vi "Keithley 6514 Read Math Result.vi"(0 "Resource In":refnum<visa-resource-name>, 1 "Check For SCPI Errors? (T)":bool=TRUE, 7 "read source (Math Result:0)":u16(ring) items=["Math Result", "Buffer Statistic"], 11 "error in (no error)":T1) -> (4 "Resource Out (dupl)":refnum<visa-resource-name>, 8 "result":dbl format="%.6e", 15 "error out":T1)   [LabVIEW 2014, in "KE6514Driver.lvlib"]
doc: "This VI is used to read the results of the selected calculation. The calculations are configured using the Math, or Buffer Math VI's. \n\nThese calculations do not show up in the other read VI's.\n\nRead Source:\n0 = Math\n1 = Buffer Math"
uses:
  KE6514Driver.lvlib
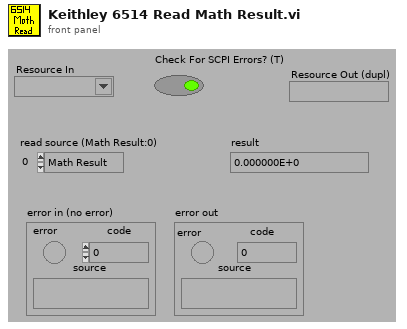
[diagram p1: front panel]
types:
  T1 = cluster{"error":bool, "code":i32, "source":string}
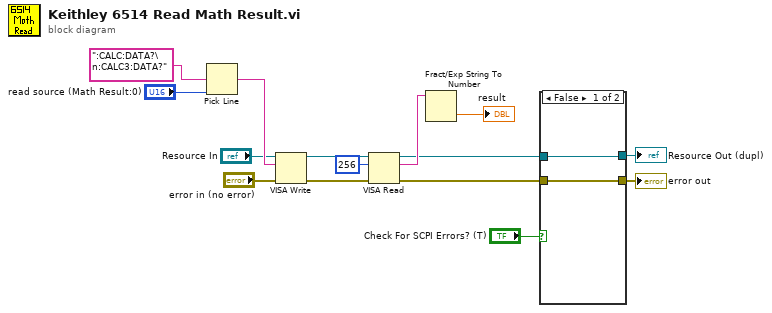
[diagram p0: block diagram]
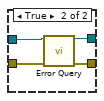
[diagram p2: hidden frame]
diagram:
  n1 = Pick Line(multi-line string=":CALC:DATA?\n:CALC3:DATA?", line index="read source (Math Result:0)") -> (output string=w8:string)  [unwired: 1 in]
  n2 = VISA Write(VISA resource name="Resource In", write buffer=w8, error in (no error)="error in (no error)") -> (VISA resource name out=w10:refnum<visa-resource-name>, error out=w11:errorcluster)  [unwired: 1 out]
  n3 = VISA Read(VISA resource name=w10, byte count=u32 256, error in (no error)=w11) -> (VISA resource name out=w4:refnum<visa-resource-name>, read buffer=w6:string, error out=w3:errorcluster)  [unwired: 1 out]
  n4 = Fract/Exp String To Number(string=w6) -> (number=→"result":dbl)  [unwired: 3 in, 1 out]
  n5 = case shown="False" "Check For SCPI Errors? (T)" {
    tunnel: w4 -> [w17 w20]
    tunnel: w3 -> [w16 w21]
    tunnel: [w16 w19] -> w1
    tunnel: [w17 w18] -> w2
    frame False {
    }
    frame True {
      n6 = call "Error Query.vi"("VISA Resource In"=w20, "error in (no error)"=w21) -> ("VISA Resource Out (dupl)"=w18:refnum<visa-resource-name>, "error out"=w19:errorcluster)  [unwired: 10 in, 2 out]
    }
  }
  "error out" <- w1
  "Resource Out (dupl)" <- w2
